vi "Tokens to Array.vi"(8 "error in":errorcluster, 10 "starting index":i32, 11 "array w/ subset deleted":cluster{"Token Type":T1, "Token Value":string}[](array[cluster])) -> (0 "error out":errorcluster, 2 "next index":i32, 3 "JSON Array out":refnum<class "JSON Array.lvclass">)   [LabVIEW 2017, in "LVJSON.lvlib"]
uses:
  LVJSON.lvlib
  JSON Data Classes/JSON Array/JSON Array.lvclass
  C:/Users/tblair/Documents/Git Projects/LVJSON/JSON Data Classes/JSON Datatype/JSON Datatype.lvclass
  Token Types.ctl
  JSON Data Classes/JSON Object/JSON Object.lvclass
  JSON Data Classes/JSON Numeric/JSON Numeric.lvclass
  JSON Data Classes/JSON Boolean/JSON Boolean.lvclass
  JSON Data Classes/JSON Null/JSON Null.lvclass
  JSON Data Classes/JSON String/JSON String.lvclass
  JSON Data Classes/JSON Numeric/New JSON Numeric.vi
  JSON Data Classes/JSON Boolean/New JSON Boolean.vi
  JSON Data Classes/JSON Null/New JSON Null.vi
  JSON Data Classes/JSON String/New JSON String.vi
  JSON Data Classes/JSON Array/New JSON Array (JSON Data).vi
  JSON Data Classes/JSON Datatype/JSON Datatype.lvclass
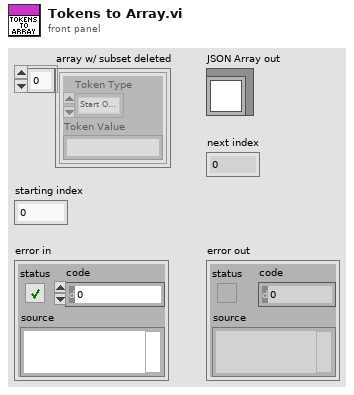
[diagram p1: front panel]
types:
  T1 = typedef "Token Types.ctl" = enum32{"Start Object", "End Object", "Start Array", "End Array", "Colon", "Comma", "Numeric", "true", "false", "null", "String"}
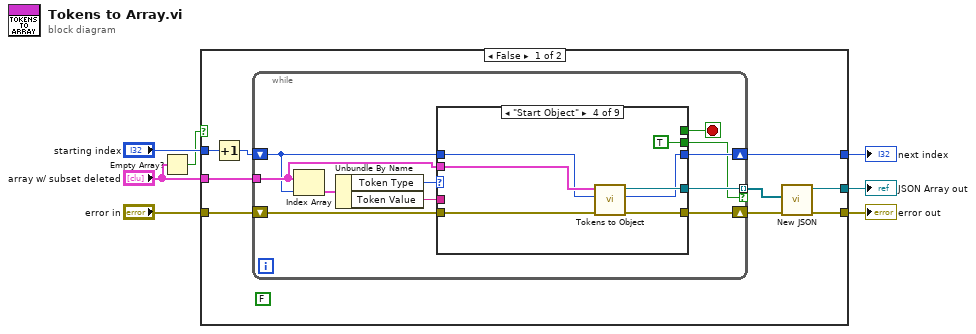
[diagram p0: block diagram]
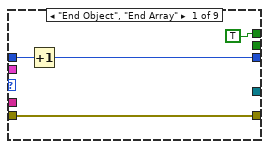
[diagram p2: hidden frame]
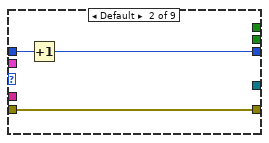
[diagram p3: hidden frame]
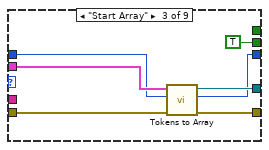
[diagram p4: hidden frame]
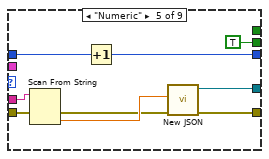
[diagram p5: hidden frame]
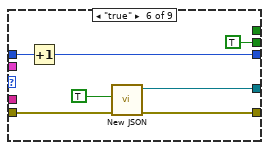
[diagram p6: hidden frame]
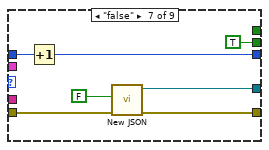
[diagram p7: hidden frame]
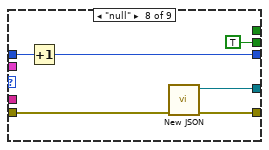
[diagram p8: hidden frame]
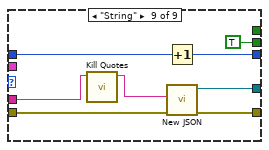
[diagram p9: hidden frame]
diagram:
  n1 = Empty Array?(array="array w/ subset deleted") -> (empty?=w1:bool)
  n2 = case shown="False" w1 {
    tunnel: [w8 _] -> w7
    tunnel: "array w/ subset deleted" -> [w16 _]
    tunnel: "error in" -> [w15 w86]
    tunnel: [w13 w86] -> w5
    tunnel: [w11 w87] -> w4
    tunnel: "starting index" -> [w10 w87]
    frame False {
      (unwired) FALSE
      n3 = Increment(x=w10) -> (x+1=w12:i32)
      n4 = while {
        tunnel: w16 -> [w20]
        tunnel: [w24] -> w9 mode=indexing if=w17
        shift-right: [w19] -> w11
        shift-left: w12 -> [w18]
        shift-right: [w21] -> w14
        shift-left: w15 -> [w22]
        stop <- w25 stop-if-true
        n5 = Index Array(array=w20, index=w18) -> (element=w23:cluster{"Token Type":T1, "Token Value":string})
        n6 = Unbundle By Name(w23) -> ("Token Type"=w27:T1, "Token Value"=w26:string)
        n7 = case shown="\"Start Object\"" w27 {
          tunnel: w26 -> [_ _ _ _ w56 _ _ _ w79]
          tunnel: [TRUE _ _ _ _ _ _ _ _] -> w25
          tunnel: [_ _ w38 w45 w57 w63 w70 w77 w85] -> w24
          tunnel: [_ _ TRUE TRUE TRUE TRUE TRUE TRUE TRUE] -> w17
          tunnel: w22 -> [w31 w34 w41 w48 w53 w61 w68 w75 w80]
          tunnel: [w31 w34 w40 w47 w51 w60 w67 w74 w84] -> w21
          tunnel: w20 -> [_ _ w39 w46 _ _ _ _ _]
          tunnel: w18 -> [w30 w33 w35 w42 w50 w59 w66 w73 w83]
          tunnel: [w29 w32 w36 w43 w49 w58 w65 w72 w82] -> w19
          frame "End Object", "End Array" {
            n8 = Increment(x=w30) -> (x+1=w29:i32)
          }
          frame Default {
            n9 = Increment(x=w33) -> (x+1=w32:i32)
          }
          frame "Start Array" {
            n10 = call "Tokens to Array.vi"("error in"=w41, "starting index"=w35, "array w/ subset deleted"=w39) -> ("error out"=w40:errorcluster, "next index"=w36:i32, "JSON Array out"=w38:refnum<class "JSON Array.lvclass">)  [unwired: 6 in]
          }
          frame "Start Object" {
            n11 = call "Tokens to Object.vi"("error in"=w48, "starting index"=w42, "array w/ subset deleted"=w46) -> ("error out"=w47:errorcluster, "next index"=w43:i32, "JSON Object out"=w45:refnum<class "JSON Object.lvclass">)  [unwired: 6 in]
          }
          frame "Numeric" {
            n12 = Scan From String(input string=w56, error in=w53) -> (error out=w52:errorcluster, output 1=w55:dbl)  [unwired: 3 in, 2 out]
            n13 = Increment(x=w50) -> (x+1=w49:i32)
            n14 = call-poly "New JSON.vi"("error in (no error)"=w52, "value"=w55) -> ("error out"=w51:errorcluster, "JSON String out"=w57:refnum<class "JSON Numeric.lvclass">)  [unwired: 8 in]
          }
          frame "true" {
            n15 = Increment(x=w59) -> (x+1=w58:i32)
            n16 = call-poly "New JSON.vi"("error in (no error)"=w61, "value"=TRUE) -> ("error out"=w60:errorcluster, "JSON String out"=w63:refnum<class "JSON Boolean.lvclass">)  [unwired: 8 in]
          }
          frame "false" {
            n17 = Increment(x=w66) -> (x+1=w65:i32)
            n18 = call-poly "New JSON.vi"("error in (no error)"=w68, "value"=FALSE) -> ("error out"=w67:errorcluster, "JSON String out"=w70:refnum<class "JSON Boolean.lvclass">)  [unwired: 8 in]
          }
          frame "null" {
            n19 = Increment(x=w73) -> (x+1=w72:i32)
            n20 = call-poly "New JSON.vi"("error in (no error)"=w75) -> ("error out"=w74:errorcluster, "JSON String out"=w77:refnum<class "JSON Null.lvclass">)  [unwired: 9 in]
          }
          frame "String" {
            n21 = call "Kill Quotes.vi"("Token Value in"=w79) -> ("Token Value out"=w78:string)  [unwired: 10 in]
            n22 = Increment(x=w83) -> (x+1=w82:i32)
            n23 = call-poly "New JSON.vi"("error in (no error)"=w80, "value"=w78) -> ("error out"=w84:errorcluster, "JSON String out"=w85:refnum<class "JSON String.lvclass">)  [unwired: 8 in]
          }
        }
      }
      n24 = call-poly "New JSON.vi"("error in (no error)"=w14, "Boolean Array"=w9) -> ("error out"=w13:errorcluster, "JSON Array out"=w8:refnum<class "JSON Array.lvclass">)  [unwired: 8 in]
    }
    frame True {
    }
  }
  "next index" <- w4
  "JSON Array out" <- w7
  "error out" <- w5
